vi "Host-FIXParser-Deserialize-Results.vi"(11 "Data in":u64[](array[numeric]) format="%.0x") -> (3 "Array":T1(array[cluster]))   [LabVIEW 2020]
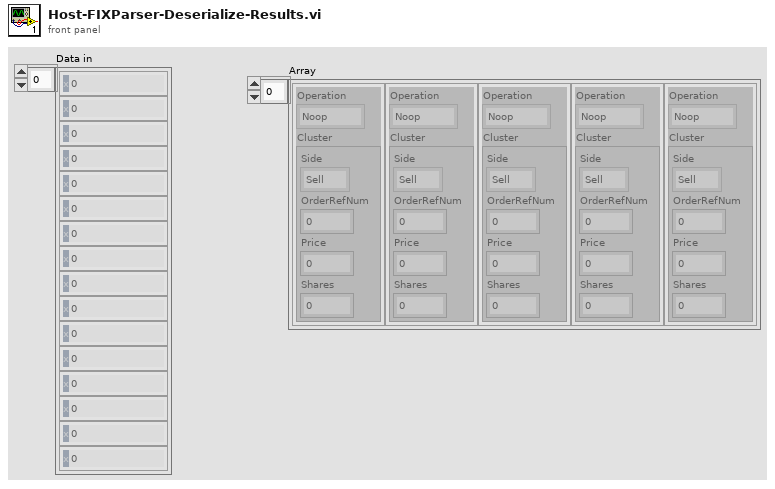
[diagram p1: front panel]
types:
  T1 = cluster{"Operation":enum16{"Noop", "GetAll", "AddOrder", "DeleteOrder"}, "Cluster":cluster{"Side":enum16{"Sell", "Buy"}, "OrderRefNum":u64, "Price":u32, "Shares":u32}}[]
  T2 = cluster{"Operation":enum16{"Noop", "GetAll", "AddOrder", "DeleteOrder"}, "Cluster":cluster{"Side":enum16{"Sell", "Buy"}, "OrderRefNum":u64, "Price":u32, "Shares":u32}}
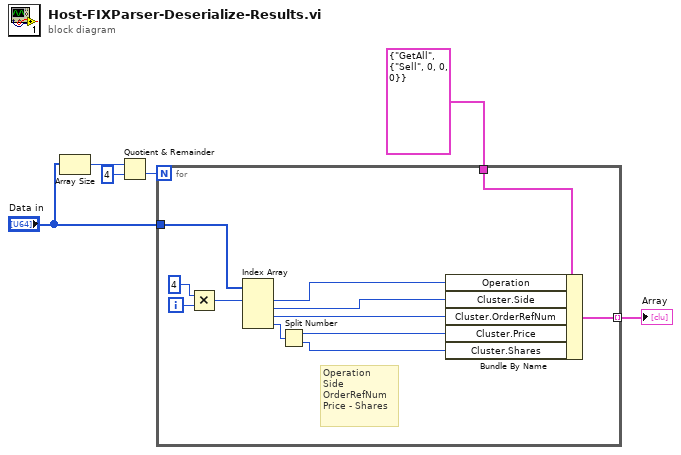
[diagram p0: block diagram]
diagram:
  n1 = Array Size(array="Data in") -> (size(s)=w6:i32)
  n2 = Quotient & Remainder(x=w6, y=4) -> (floor(x/y)=w4:i32)  [unwired: 1 out]
  n3 = for {
    N: w4 -> [_]
    tunnel: T2 {"Operation"=enum."GetAll", "Cluster"={"Side"=enum."Sell", "OrderRefNum"=0, "Price"=0, "Shares"=0}} ("OrderBookCommand") -> [w13]
    tunnel: [w14] -> w1 mode=indexing
    tunnel: "Data in" -> [w16]
    i -> [w18]
    # "Operation\nSide\nOrderRefNum\nPrice - Shares"
    n4 = Multiply(x=4, y=w18) -> (x*y=w15:i32)
    n5 = Index Array(array=w16, index #1=w15) -> (element #1=w12:u64, element #2=w7:u64, element #3=w11:u64, element #4=w10:u64)  [unwired: 3 in]
    n6 = Split Number(x=w10) -> (hi(x)=w9:u32, lo(x)=w8:u32)
    n7 = Bundle By Name(cluster=w13, "Operation"=w12, "Cluster.Side"=w7, "Cluster.OrderRefNum"=w11, "Cluster.Price"=w9, "Cluster.Shares"=w8) -> (w14:T2)
  }
  "Array" <- w1
